vi "templogger.vi"() -> ()   [LabVIEW 2015]
doc: "This VI is a solution to an exercise in the LabVIEW Basics I course.\n\nThis VI continuously acquires and calculates a 3-point running average of the temperature. If ANALYSIS is on, the VI will calculate the high value, and turn on a Warning LED if the temperature passes a high limit."
panel:
  in  "analyze":bool=TRUE
  in  "?":bool=TRUE
  out "High Value":dbl
  out "?":cluster{dbl, "Temperature":dbl}(graph)
  out "Warning":bool
  in  "High Limit":dbl=80.0 format="%.2f"
  # "ON\n\nOFF"
  # "ON\n\nOFF"
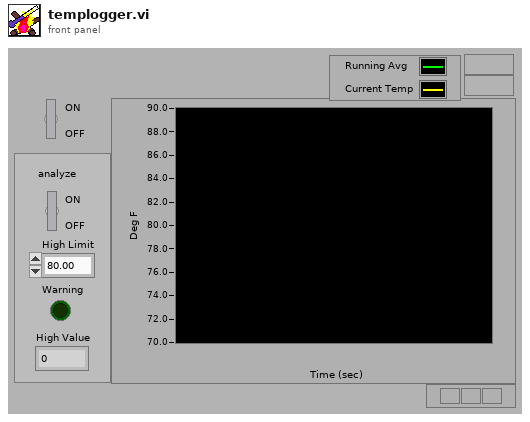
[diagram p1: front panel]
types:
  T1 = enum16{"open", "open or create", "create or replace", "create", "open (read only)"}
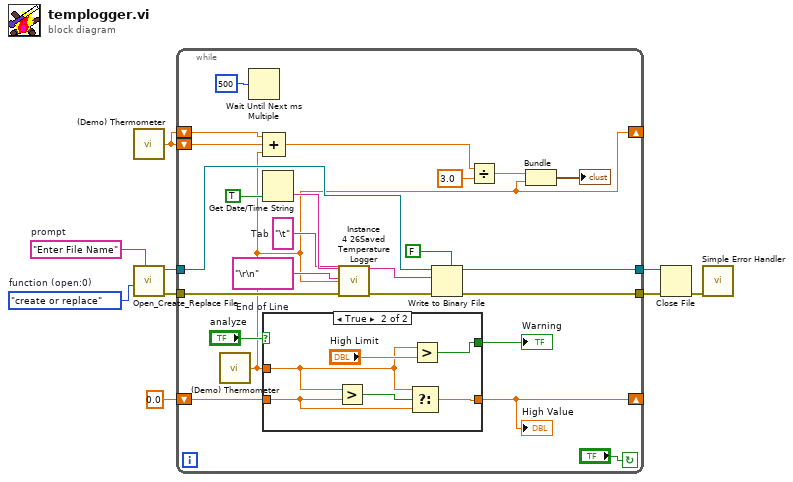
[diagram p0: block diagram]
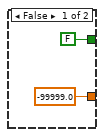
[diagram p2: hidden frame]
diagram:
  w1 = T1."create or replace"  # function (open:0)
  w2 = "Enter File Name"  # prompt
  n1 = call "(Demo) Thermometer.vi"() -> ("Temperature"=w9:dbl)  [unwired: 1 in]
  n2 = call <vilib>:"Open_Create_Replace File.vi"("prompt"=w2, "function (open:0)"=w1) -> ("error out"=w3:errorcluster, "refnum"=w7:refnum<file>)  [unwired: 6 in, 2 out]
  n3 = while {
    shift-left: w9 -> [w29]
    shift-left: w9 -> [w30]
    shift-right: [w12] -> _
    shift-right: [w25] -> _
    shift-left: 0.0 -> [w26]
    tunnel: w7 -> [w21]
    tunnel: [w20] -> w6
    tunnel: [w19] -> w5
    tunnel: w3 -> [w17]
    stop <- "?" continue-if-true
    w13 = "\r\n"  # End of Line
    w14 = "\t"  # Tab
    n4 = call "(Demo) Thermometer.vi"() -> ("Temperature"=w12:dbl)  [unwired: 1 in]
    n5 = Wait Until Next ms Multiple(millisecond multiple=u32 500) -> ()  [unwired: 1 out]
    n6 = Compound Arithmetic op=ADD(w30, w29, w12) -> (w28:dbl)
    n7 = Get Date/Time String(want seconds? (F)=TRUE) -> (time string=w16:string)  [unwired: 2 in, 1 out]
    n8 = case shown="True" "analyze" {
      tunnel: w12 -> [_ w40]
      tunnel: w26 -> [_ w39]
      tunnel: [-99999.0 ("Temperature") w37] -> w25
      tunnel: [FALSE w36] -> w24
      frame False {
      }
      frame True {
        n9 = Greater?(x=w40, y=w39) -> (0:w38:bool)
        n10 = Select(t=w40, s=w38, f=w39) -> (s? t:f=w37:dbl)
        n11 = Greater?(x=w40, y="High Limit") -> (0:w36:bool)
      }
    }
    "Warning" <- w24
    "High Value" <- w25
    n12 = call "Instance           4 26Saved   Temperature Logger .vi"("Beginning Text"=w16, "tab"=w14, "temp"=w12, "end"=w13, "error in (no error)"=w17) -> ("Result"=w11:string, "error out"=w18:errorcluster)  [unwired: 9 in]
    n13 = Write to Binary File(file (use dialog)=w21, data=w11, error in=w18, 5:FALSE ("prepend array or string size? (T)")) -> (refnum out=w20:refnum<file>, error out=w19:errorcluster)  [unwired: 2 in, 1 out]
    n14 = Divide(x=w28, y=3.0) -> (x/y=w31:dbl)
    n15 = Bundle "Bundle"(w31, "Temperature"=w12) -> (→"?":cluster{dbl, "Temperature":dbl})  [unwired: 1 in]
  }
  n16 = Close File(refnum=w6, error in=w5) -> (error out=w4:errorcluster)  [unwired: 1 out]
  n17 = call <vilib>:"Simple Error Handler.vi"("error in (no error)"=w4) -> ()  [unwired: 4 in, 5 out]
